vi "Reserve Method.vi"(8 "error in (no error)":errorcluster, 11 "LUnit Test Case In":refnum<class "LUnit Test Case.lvclass">) -> (0 "error out":errorcluster, 3 "LUnit Test Case Out":refnum<class "LUnit Test Case.lvclass">)   [LabVIEW 2020, in "LUnit Test Case.lvclass"]
uses:
  LUnit Test Case.lvclass
  LUnit Test Case.lvclass/LUnit Test Case.ctl
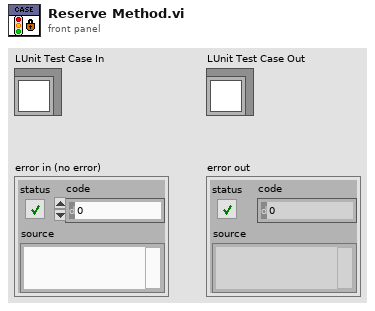
[diagram p1: front panel]
types:
  T1 = typedef "Semaphore RefNum" = refnum<k1>
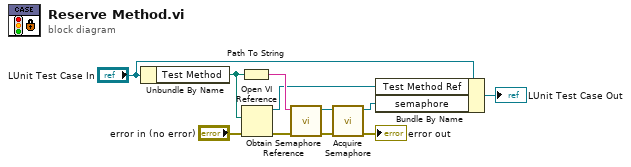
[diagram p0: block diagram]
diagram:
  n1 = Unbundle By Name("LUnit Test Case In") -> ("Test Method"=w4:path)
  n2 = Path To String(path=w4) -> (string=w10:string)
  n3 = Open VI Reference(vi path=w4, error in (no error)="error in (no error)") -> (vi reference=w2:refnum<vi>, error out=w9:errorcluster)  [unwired: 4 in]
  n4 = call <vilib>:"Obtain Semaphore Reference.vi"("error in (no error)"=w9, "name (unnamed)"=w10) -> ("error out"=w8:errorcluster, "semaphore"=w6:T1)  [unwired: 3 in, 1 out]
  n5 = call <vilib>:"Acquire Semaphore.vi"("error in (no error)"=w8, "semaphore"=w6) -> ("error out"=→"error out":errorcluster, "semaphore out"=w1:T1)  [unwired: 3 in, 1 out]
  n6 = Bundle By Name(cluster="LUnit Test Case In", "Test Method Ref"=w2, "semaphore"=w1) -> (→"LUnit Test Case Out":refnum<class "LUnit Test Case.lvclass">)
